vi "test-swerve-drive-kinematics-12.vi"() -> (3 "Test Passed":bool)   [LabVIEW 2019]
uses:
  <vilib>/Rock Robotics/WPI/ThirdParty/JAS_Junk/TrajLib/Trajectory_Library.lvlib
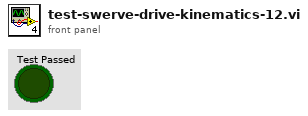
[diagram p1: front panel]
types:
  T1 = typedef "Trajectory_Library.lvlib/TRANSLATION2D.ctl" = cluster{"X":dbl, "Y":dbl}
  T2 = typedef "Trajectory_Library.lvlib/SWERVE_DRIVE_KINEMATICS.ctl" = cluster{"NumModules":i32, "InverseKinematics":T3, "ForwardKinematics":T3, "Modules":T1[], "PrevCoR":T1, "SavedModuleStates":T4[]}
  T3 = typedef "NI_Matrix.lvlib/RealMatrix.ctl" = dbl[][]
  T4 = typedef "Trajectory_Library.lvlib/SWERVE_DRIVE_MODULE_STATE.ctl" = cluster{"Speed":dbl, "Angle":T5}
  T5 = typedef "Trajectory_Library.lvlib/ROTATION2D.ctl" = cluster{"VALUE":dbl, "COS":dbl, "SIN":dbl}
  T6 = typedef "Trajectory_Library.lvlib/CHASSIS_SPEEDS.ctl" = cluster{"vX":dbl, "vY":dbl, "vOmega":dbl}
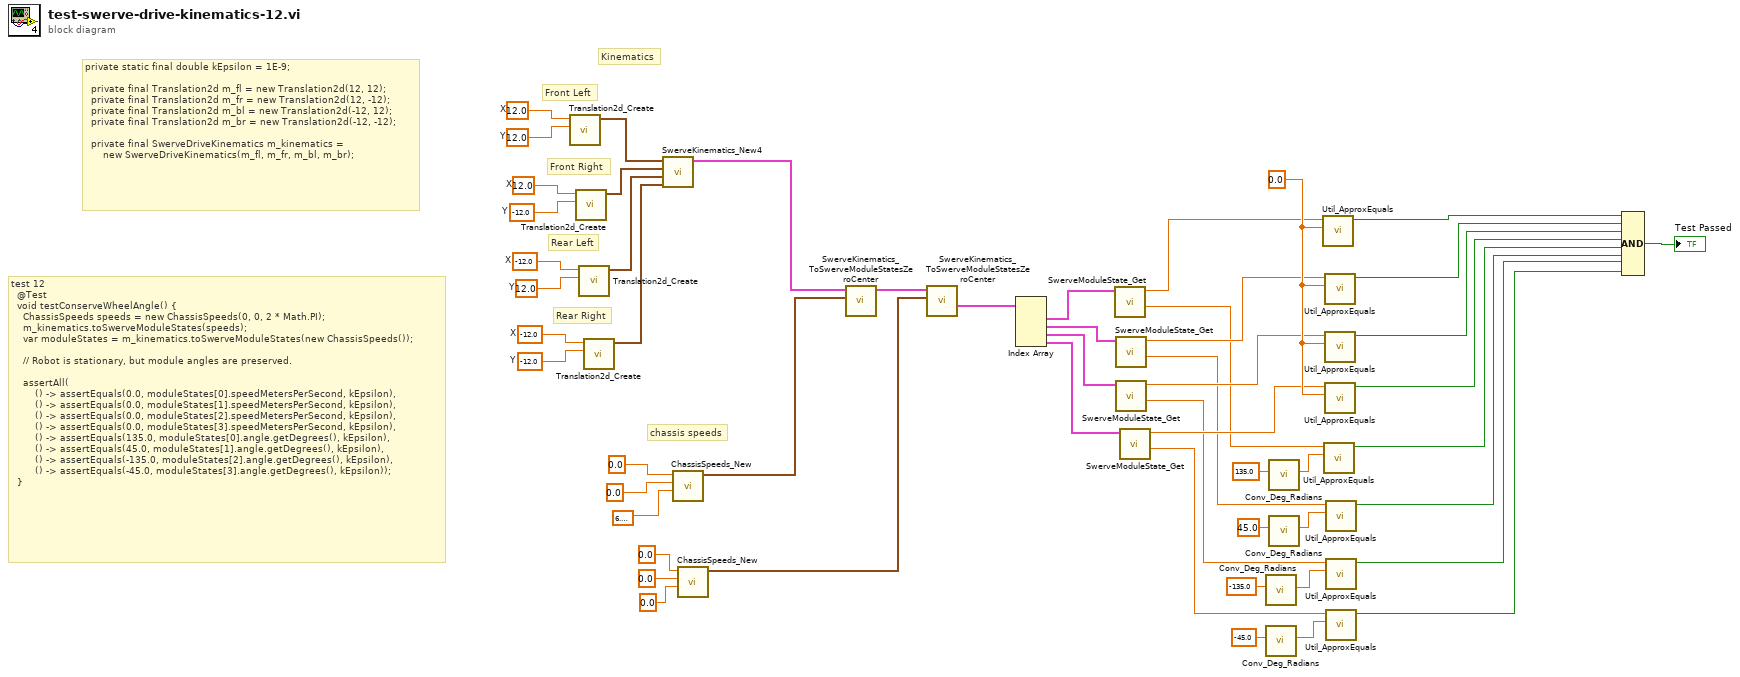
[diagram p0: block diagram]
diagram:
  w28 = 0.0 ("Value 2")
  w45 = -12.0  # X
  w44 = -12.0  # Y
  w43 = -12.0  # X
  w42 = 12.0  # Y
  w41 = 12.0  # X
  w40 = -12.0  # Y
  w39 = 12.0  # X
  w38 = 12.0  # Y
  # "Kinematics"
  # "Rear Right"
  # "Rear Left"
  # "Front Right"
  # "Front Left"
  # "chassis speeds"
  # "private static final double kEpsilon = 1E-9;\n\n  private final Translation2d m_fl = new Translation2d(12, 12);\n  private final Translation2d m_fr = new Translation2d(12, -12);\n  private final Translation2d m_bl = new Translation2d(-12, 12);\n  private final Translation2d m_br = new Translation2d(-12, -12);\n\n  private final SwerveDriveKinematics m_kinematics =\n      new SwerveDriveKinematics(m_fl, m_fr, m_bl, m_br);"
  # "test 12\n  @Test  \n  void testConserveWheelAngle() {\n    ChassisSpeeds speeds = new ChassisSpeeds(0, 0, 2 * Math.PI);\n    m_kinematics.toSwerveModuleStates(speeds);\n    var moduleStates = m_kinematics.toSwerveModuleStates(new ChassisSpeeds());\n\n    // Robot is stationary, but module angles are preserved.\n\n    assertAll(\n        () -> assertEquals(0.0, moduleStates[0].speedMetersPerSecond, kEpsilon),\n        () -> assertEquals(0.0, moduleStates[1].speedMetersPerSecond, kEpsilon),\n        () -> assertEquals(0.0, moduleStates[2].speedMetersPerSecond, kEpsilon),\n        () -> assertEquals(0.0, moduleStates[3].speedMetersPerSecond, kEpsilon),\n        () -> assertEquals(135.0, moduleStates[0].angle.getDegrees(), kEpsilon),\n        () -> assertEquals(45.0, moduleStates[1].angle.getDegrees(), kEpsilon),\n        () -> assertEquals(-135.0, moduleStates[2].angle.getDegrees(), kEpsilon),\n        () -> assertEquals(-45.0, moduleStates[3].angle.getDegrees(), kEpsilon));\n  }"
  n1 = call <vilib>:"Translation2d_Create.vi"("Y"=w38, "X"=w39) -> ("TRANSLATION"=w46:T1)  [unwired: 9 in]
  n2 = call <vilib>:"Translation2d_Create.vi"("Y"=w40, "X"=w41) -> ("TRANSLATION"=w47:T1)  [unwired: 9 in]
  n3 = call <vilib>:"Translation2d_Create.vi"("Y"=w42, "X"=w43) -> ("TRANSLATION"=w48:T1)  [unwired: 9 in]
  n4 = call <vilib>:"Translation2d_Create.vi"("Y"=w44, "X"=w45) -> ("TRANSLATION"=w49:T1)  [unwired: 9 in]
  n5 = call <vilib>:"SwerveKinematics_New4.vi"("wheel 3"=w49, "wheel 2"=w48, "wheel 1"=w47, "wheel 0"=w46) -> ("SWERVE_DRIVE_KINEMATICS"=w37:T2)  [unwired: 7 in]
  n6 = call <vilib>:"ChassisSpeeds_New.vi"("vAngular"=6.283185307179586, "vY"=0.0, "vX"=0.0) -> ("CHASSIS"=w36:T6)  [unwired: 8 in]
  n7 = call <vilib>:"ChassisSpeeds_New.vi"("vAngular"=0.0, "vY"=0.0, "vX"=0.0) -> ("CHASSIS"=w34:T6)  [unwired: 8 in]
  n8 = call <vilib>:"SwerveKinematics_ToSwerveModuleStatesZeroCenter.vi"("ChassisSpeeds"=w36, "in SWERVE_DRIVE_KINEMATICS"=w37) -> ("out SWERVE_DRIVE_KINEMATICS"=w35:T2)  [unwired: 8 in, 1 out]
  n9 = call <vilib>:"SwerveKinematics_ToSwerveModuleStatesZeroCenter.vi"("ChassisSpeeds"=w34, "in SWERVE_DRIVE_KINEMATICS"=w35) -> ("ModuleStates"=w33:T4[])  [unwired: 8 in, 1 out]
  n10 = Index Array(array=w33) -> (element #1=w32:T4, element #2=w31:T4, element #3=w30:T4, element #4=w29:T4)  [unwired: 4 in]
  n11 = call <vilib>:"SwerveModuleState_Get.vi"("Desired State"=w32) -> ("Angle RADIANS"=w23:dbl, "Speed M/S"=w27:dbl)  [unwired: 9 in]
  n12 = call <vilib>:"SwerveModuleState_Get.vi"("Desired State"=w31) -> ("Angle RADIANS"=w22:dbl, "Speed M/S"=w26:dbl)  [unwired: 9 in]
  n13 = call <vilib>:"SwerveModuleState_Get.vi"("Desired State"=w30) -> ("Angle RADIANS"=w21:dbl, "Speed M/S"=w25:dbl)  [unwired: 9 in]
  n14 = call <vilib>:"SwerveModuleState_Get.vi"("Desired State"=w29) -> ("Angle RADIANS"=w20:dbl, "Speed M/S"=w24:dbl)  [unwired: 9 in]
  n15 = call <vilib>:"Conv_Deg_Radians.vi"("Degress"=-135.0) -> ("Radians"=w18:dbl)  [unwired: 10 in]
  n16 = call <vilib>:"Conv_Deg_Radians.vi"("Degress"=-45.0) -> ("Radians"=w19:dbl)  [unwired: 10 in]
  n17 = call <vilib>:"Conv_Deg_Radians.vi"("Degress"=135.0) -> ("Radians"=w16:dbl)  [unwired: 10 in]
  n18 = call <vilib>:"Conv_Deg_Radians.vi"("Degress"=45.0) -> ("Radians"=w17:dbl)  [unwired: 10 in]
  n19 = call <vilib>:"Util_ApproxEquals.vi"("Value 2"=w28, "Value 1"=w27) -> ("ApproxEquals"=w11:bool)  [unwired: 9 in]
  n20 = call <vilib>:"Util_ApproxEquals.vi"("Value 2"=w16, "Value 1"=w23) -> ("ApproxEquals"=w7:bool)  [unwired: 9 in]
  n21 = call <vilib>:"Util_ApproxEquals.vi"("Value 2"=w28, "Value 1"=w26) -> ("ApproxEquals"=w10:bool)  [unwired: 9 in]
  n22 = call <vilib>:"Util_ApproxEquals.vi"("Value 2"=w28, "Value 1"=w25) -> ("ApproxEquals"=w9:bool)  [unwired: 9 in]
  n23 = call <vilib>:"Util_ApproxEquals.vi"("Value 2"=w28, "Value 1"=w24) -> ("ApproxEquals"=w8:bool)  [unwired: 9 in]
  n24 = call <vilib>:"Util_ApproxEquals.vi"("Value 2"=w17, "Value 1"=w22) -> ("ApproxEquals"=w6:bool)  [unwired: 9 in]
  n25 = call <vilib>:"Util_ApproxEquals.vi"("Value 2"=w18, "Value 1"=w21) -> ("ApproxEquals"=w5:bool)  [unwired: 9 in]
  n26 = call <vilib>:"Util_ApproxEquals.vi"("Value 2"=w19, "Value 1"=w20) -> ("ApproxEquals"=w4:bool)  [unwired: 9 in]
  n27 = Compound Arithmetic op=AND(w11, w10, w9, w8, w7, w6, w5, w4) -> (→"Test Passed":bool)
